vi "pid.vi"(1 "y":dbl, 2 "Kp":dbl, 3 "Te":dbl, 4 "r-Set point":dbl, 5 "Kd":dbl, 6 "Ki":dbl) -> (0 "u":dbl)   [LabVIEW 2010]
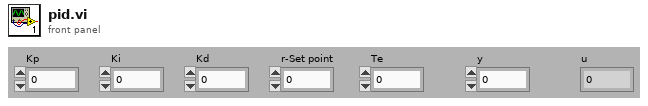
[diagram p1: front panel]
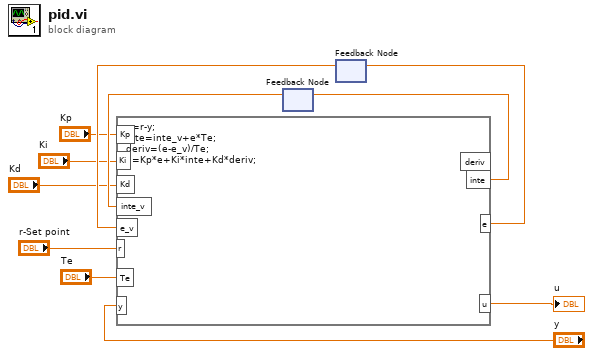
[diagram p0: block diagram]
diagram:
  n1 = feedback #1() -> (w5:dbl)  [unwired: 1 in]
  n2 = feedback #2() -> (w7:dbl)  [unwired: 1 in]
  n3 = formula code="e=r-y;\ninte=inte_v+e*Te;\nderiv=(e-e_v)/Te;\nu=Kp*e+Ki*inte+Kd*deriv;"("Kp"="Kp", "Ki"="Ki", "Kd"="Kd", "inte_v"=w5, "e_v"=w7, "r"="r-Set point", "Te"="Te", "y"="y") -> ("inte"=w4:dbl, "e"=w6:dbl, "u"=→"u":dbl)  [unwired: 1 out]
  n4 = feedback-in #1(w4) -> ()
  n5 = feedback-in #2(w6) -> ()
